vi "Get Strings from Ref.vi"(8 "error in (no error)":errorcluster, 9 "Label Prefix":string, 10 "GObj Refnum in":refnum<vi>, 11 "FPTitle in":refnum<class "FrontPanel.lvclass">) -> (0 "error out":errorcluster, 1 "Valid?":bool, 2 "GObj Refnum out":refnum<vi>, 3 "FPTitle out":refnum<class "FrontPanel.lvclass">, 4 "GObj Name":string)   [LabVIEW 2013, in "SET Project Data.lvlib" / "FrontPanel.lvclass"]
uses:
  FrontPanel.lvclass
  GObject/GObject.lvclass/GObject.ctl
  GObject/Write UID.vi
  GObject/Write ClassName.vi
  GObject/Write Label.vi
  GObject/GObject.lvclass
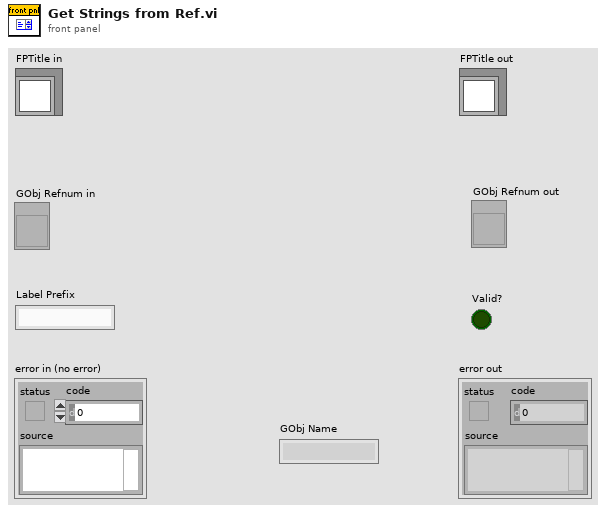
[diagram p1: front panel]
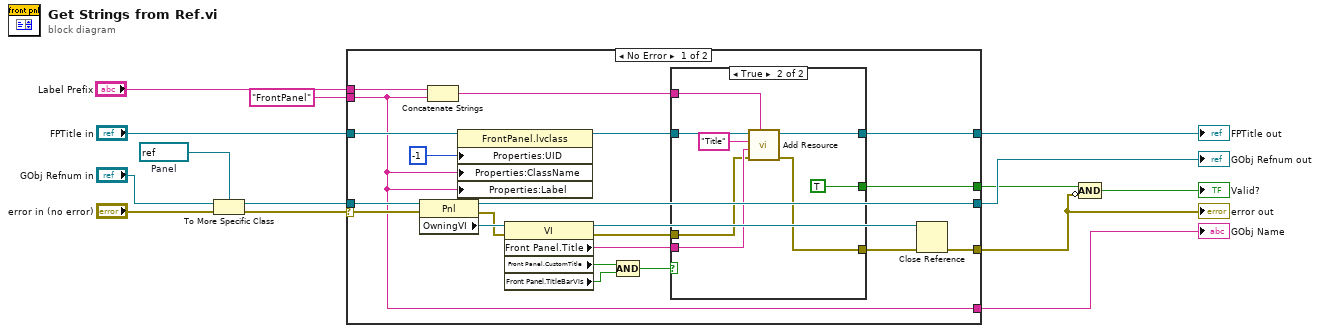
[diagram p0: block diagram]
diagram:
  w13 = refnum<vi> refnum  # Panel
  n1 = To More Specific Class(target class=w13, reference="GObj Refnum in", error in="error in (no error)") -> (specific class reference=w9:refnum<vi>, error out=w11:errorcluster)
  n2 = case shown="No Error" w11 {
    selector: w11 -> [w31 w47]
    tunnel: "FPTitle in" -> [w35 w49]
    tunnel: w9 -> [w32 w48]
    tunnel: "Label Prefix" -> [w22 _]
    tunnel: [w19 w49] -> w7
    tunnel: [w24 w48] -> w6
    tunnel: [w23 w47] -> w2
    tunnel: [w20 w46] -> w5
    tunnel: "FrontPanel" ("ClassName") -> [w20 w46]
    tunnel: [w15 _] -> w3
    frame No Error {
      n3 = property class="Pnl"(reference=w32, error in=w31) -> (reference out=w24:refnum<vi>, error out=w27:errorcluster, "OwningVI"=w30:refnum<vi>)
      n4 = Concatenate Strings(w22, w20) -> (w21:string)
      n5 = property class="FrontPanel.lvclass"(reference=w35, "Properties:UID"=-1 ("UID"), "Properties:ClassName"=w20, "Properties:Label"=w20) -> (reference out=w33:refnum<class "FrontPanel.lvclass">)  [unwired: 1 in, 1 out]
      n6 = property class="VI"(reference=w30, error in=w27) -> (reference out=w28:refnum<vi>, error out=w26:errorcluster, "Front Panel.Title"=w29:string, "Front Panel.CustomTitle"=w18:bool, "Front Panel.TitleBarVis"=w17:bool)
      n7 = Compound Arithmetic op=AND(w18, w17) -> (w16:bool)
      n8 = case shown="True" w16 {
        tunnel: w33 -> [w37 w44]
        tunnel: w29 -> [_ w43]
        tunnel: w26 -> [w36 w42]
        tunnel: [w36 w41] -> w25
        tunnel: w21 -> [_ w40]
        tunnel: [w37 w39] -> w19
        tunnel: [_ TRUE] -> w15
        frame False {
        }
        frame True {
          n9 = call "Add Resource.vi"("TagPrefix"=w40, "error in (no error)"=w42, "ItemText"=w43, "ItemName"="Title", "GObject in"=w44) -> ("error out"=w41:errorcluster, "GObject out"=w39:refnum<class "FrontPanel.lvclass">)  [unwired: 5 in]
        }
      }
      n10 = Close Reference(reference=w28, error in (no error)=w25) -> (error out=w23:errorcluster)
    }
    frame Error {
    }
  }
  "error out" <- w2
  "FPTitle out" <- w7
  "GObj Refnum out" <- w6
  "GObj Name" <- w5
  n11 = Compound Arithmetic op=AND(w3, invert w2) -> (→"Valid?":bool)
